vi "FwdKin.vi"(11 "L":dbl) -> (0 "x":T1, 2 "theta":dbl, 3 "r":dbl)   [LabVIEW 2019]
uses:
  <vilib>/Analysis/Matrix/Datatypes/RealMatrix.ctl
  <vilib>/Analysis/Matrix/NI_Matrix.lvlib
panel:
  in  "q":dbl[](array[numeric])
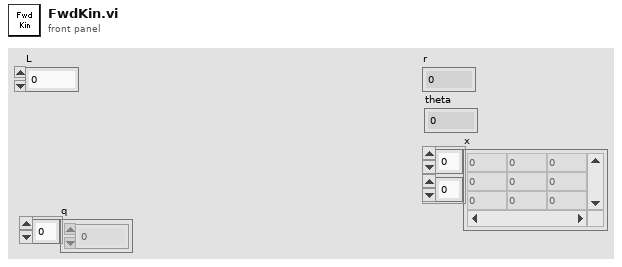
[diagram p1: front panel]
types:
  T1 = typedef "NI_Matrix.lvlib/RealMatrix.ctl" = dbl[][]
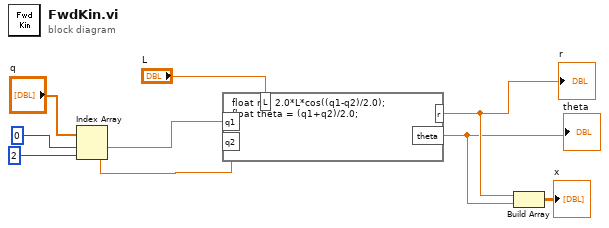
[diagram p0: block diagram]
diagram:
  n1 = Index Array(array="q", index #1=0 ("index (row)"), index #2=2 ("index (col)")) -> (element #1=w2:dbl, element #2=w1:dbl)
  n2 = formula code="float r = 2.0*L*cos((q1-q2)/2.0);\nfloat theta = (q1+q2)/2.0;"("q2"=w1, "L"="L", "q1"=w2) -> ("r"=w8:dbl, "theta"=w7:dbl)
  "r" <- w8
  "theta" <- w7
  n3 = Build Array(w8, w7) -> (→"x":T1)
